vi "Copy Template Files.vi"(8 "error in (no error)":errorcluster, 11 "Base Path":path) -> (0 "error out":errorcluster)   [LabVIEW 2015]
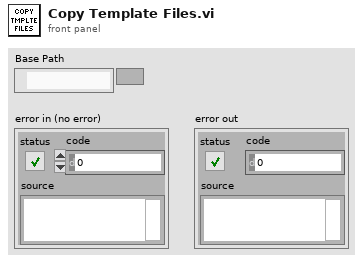
[diagram p1: front panel]
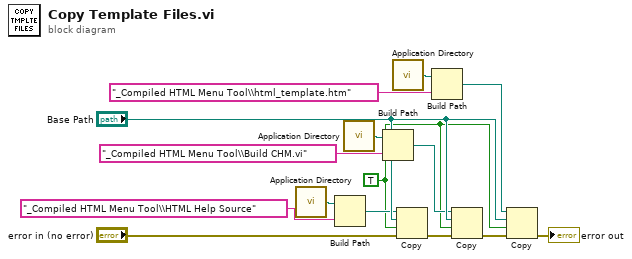
[diagram p0: block diagram]
diagram:
  w1 = TRUE ("overwrite (F)")
  n1 = call <vilib>:"Application Directory.vi"() -> ("Application Directory"=w2:path)
  n2 = Build Path(base path=w2, name or relative path="_Compiled HTML Menu Tool\\HTML Help Source") -> (appended path=w4:path)
  n3 = call <vilib>:"Application Directory.vi"() -> ("Application Directory"=w6:path)
  n4 = Build Path(base path=w6, name or relative path="_Compiled HTML Menu Tool\\Build CHM.vi") -> (appended path=w8:path)
  n5 = call <vilib>:"Application Directory.vi"() -> ("Application Directory"=w10:path)
  n6 = Copy(8:"error in (no error)", 9:w1, 10:"Base Path", 11:w4) -> (0:w9:errorcluster)  [unwired: 1 in, 2 out]
  n7 = Build Path(base path=w10, name or relative path="_Compiled HTML Menu Tool\\html_template.htm") -> (appended path=w12:path)
  n8 = Copy(8:w9, 9:w1, 10:"Base Path", 11:w8) -> (0:w13:errorcluster)  [unwired: 1 in, 2 out]
  n9 = Copy(8:w13, 9:w1, 10:"Base Path", 11:w12) -> (0:→"error out":errorcluster)  [unwired: 1 in, 2 out]
